vi "constant--init data.vi"() -> (0 "init data":T1={"state"=enum."running", "started at"=timestamp(0 s since 1904-01-01), "last resumed at"=timestamp(0 s since 1904-01-01), "last paused at"=timestamp(0 s since 1904-01-01), "total time running (seconds)"=0.0, "total time paused (seconds)"=0.0} {"total time paused (seconds)" format="%.3f"; "total time running (seconds)" format="%.3f"})   [LabVIEW 2020, in "main.lvlib" / "stopwatch_timer.lvlib"]
uses:
  stopwatch_timer.lvlib
  stopwatch data.ctl
  state.ctl
panel:
  # "Development\ncontrols/indicators useful for development and testing, but which are not outputs of the VI"
  # "Input\nInputs to the VI"
  # "Output\nOutputs of the VI"
  # "Description\n\nBlank VI with error handling case. \n\nSummarize the use of this VI in this space."
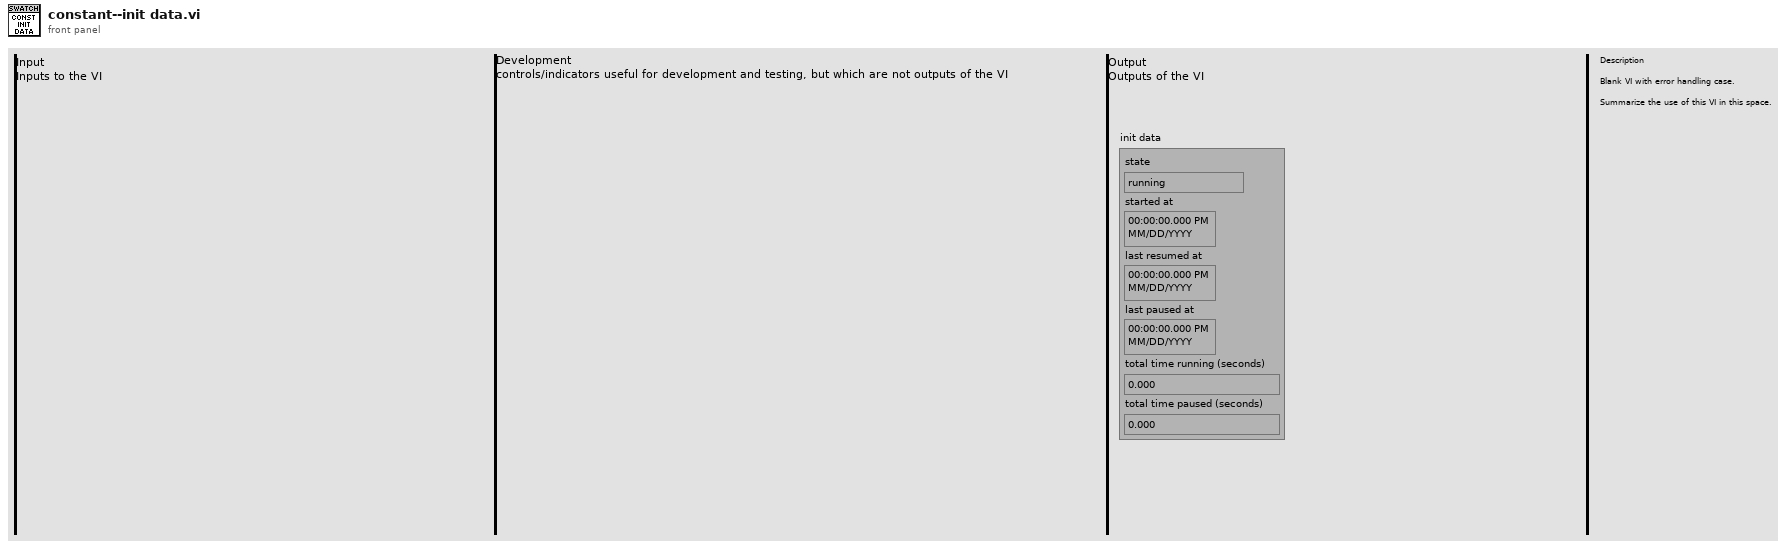
[diagram p1: front panel]
types:
  T1 = typedef "main.lvlib/stopwatch_timer.lvlib/stopwatch data.ctl" = cluster{"state":T2, "started at":timestamp, "last resumed at":timestamp, "last paused at":timestamp, "total time running (seconds)":dbl, "total time paused (seconds)":dbl}
  T2 = typedef "main.lvlib/stopwatch_timer.lvlib/state.ctl" = enum16{"not started", "running", "paused"}
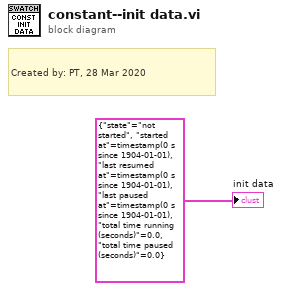
[diagram p0: block diagram]
diagram:
  # "Created by: PT, 28 Mar 2020"
  "init data" <- T1 {"state"=enum."not started", "started at"=timestamp(0 s since 1904-01-01), "last resumed at"=timestamp(0 s since 1904-01-01), "last paused at"=timestamp(0 s since 1904-01-01), "total time running (seconds)"=0.0, "total time paused (seconds)"=0.0} ("start data")
